vi "1mabsclass_1000dt.vi"() -> (0 "max jitter (uS)":dbl format="%.2f", 1 "mean time (uS)":dbl format="%.2f", 2 "standard deviation (uS)":dbl format="%.2f", 3 "execution histogram":T1(graph), 4 "Error":errorcluster, 5 "execution times (uS)":dbl[](graph))   [LabVIEW 2013]
uses:
  <vilib>/platform/TimedLoop/XDataNode/XDataNode.xnode
  <vilib>/Platform/TimedLoop/XDataNode/nitl_modes.ctl
  <vilib>/Platform/TimedLoop/XDataNode/XDNodeRunTimeDep.lvlib
  <vilib>/Platform/TimedLoop/XDataNode/wakeup.ctl
  <vilib>/Platform/TimedLoop/XDataNode/timing_clust.ctl
  absolute timing source/absolute usec timing source.lvclass
panel:
  out "act start":timestamp
  out "x-y":dbl
  out "current time":timestamp
  out "start":timestamp
  out "actual":dbl format="%#_32f"
  out "desired":dbl format="%#_32f"
  out "diff":dbl format="%#_32f"
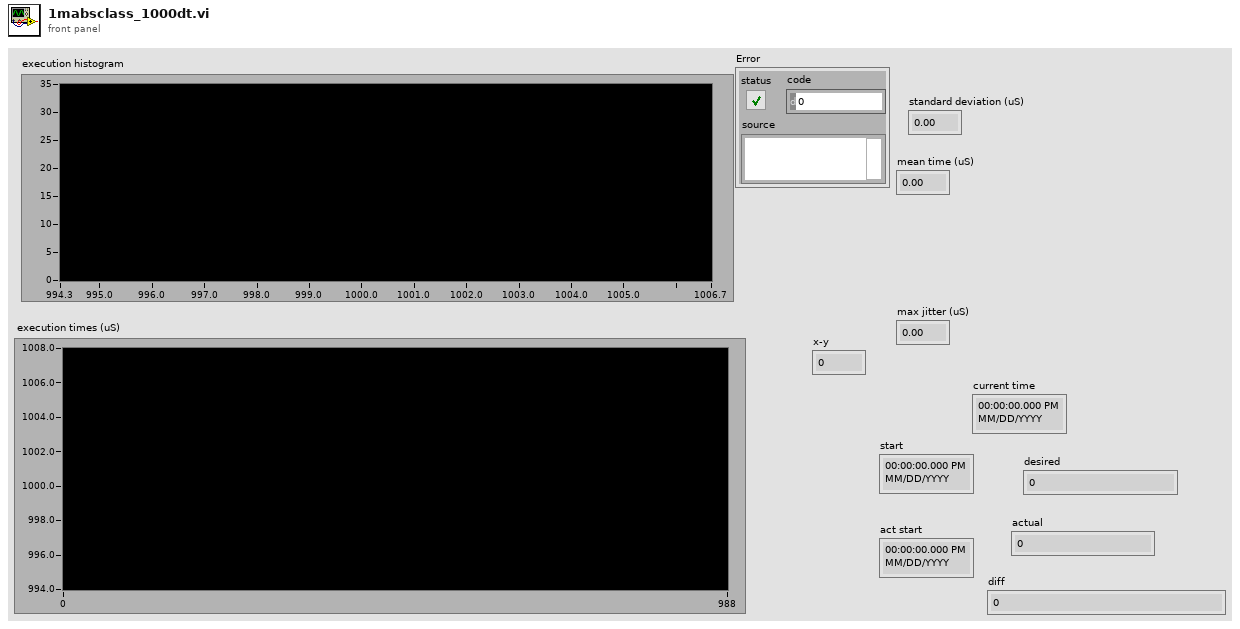
[diagram p1: front panel]
types:
  T1 = cluster{"X Values":dbl[], "Histogram: h(x)":i32[]}
  T2 = typedef "LVDateTimeRec.ctl" = cluster{"fractional second":dbl, "second":i32, "minute":i32, "hour":i32, "day of month":i32, "month":i32, "year":i32, "day of week":i32, "day of year":i32, "DST":i32}
  T3 = typedef "XDNodeRunTimeDep.lvlib/timing_clust.ctl" = cluster{"Expected End [f-1]":u64, "Actual End [f-1]":u64, "Finished Late? [f-1]":bool, "Expected End [i-1]":u64, "Actual End [i-1]":u64, "Finished Late? [i-1]":bool, "Expected Start [i]":u64, "Actual Start [i]":u64, "Expected Start [f]":u64, "Actual Start [f]":u64, "Source Name":string, "Structure Name":string, "Period":i64, "Deadline":i64, "Offset":i64, "Start":i64, "Priority":i32, "Timeout":i32, "Mode":T4, "Wakeup Reason":T5, "Error":errorcluster, "Source Type":string, "Secondary Source Type":string, "Global End Time":u64, "Global Start Time":u64, "Frame Duration":u64, "Iteration Duration":u64, "Assigned CPU":i32, "I/O Scan Engine Mode":u32}
  T4 = typedef "XDNodeRunTimeDep.lvlib/nitl_modes.ctl" = enum32{"No Change", "Process missed periods, maintain original phase", "Discard missed periods, maintain original phase", "Process missed periods, ignore original phase", "Discard missed periods, ignore original phase"}
  T5 = typedef "XDNodeRunTimeDep.lvlib/wakeup.ctl" = enum32{"Normal", "Aborted", "Asynchronous wakeup", "Timing source error", "Timed loop error", "Timeout"}
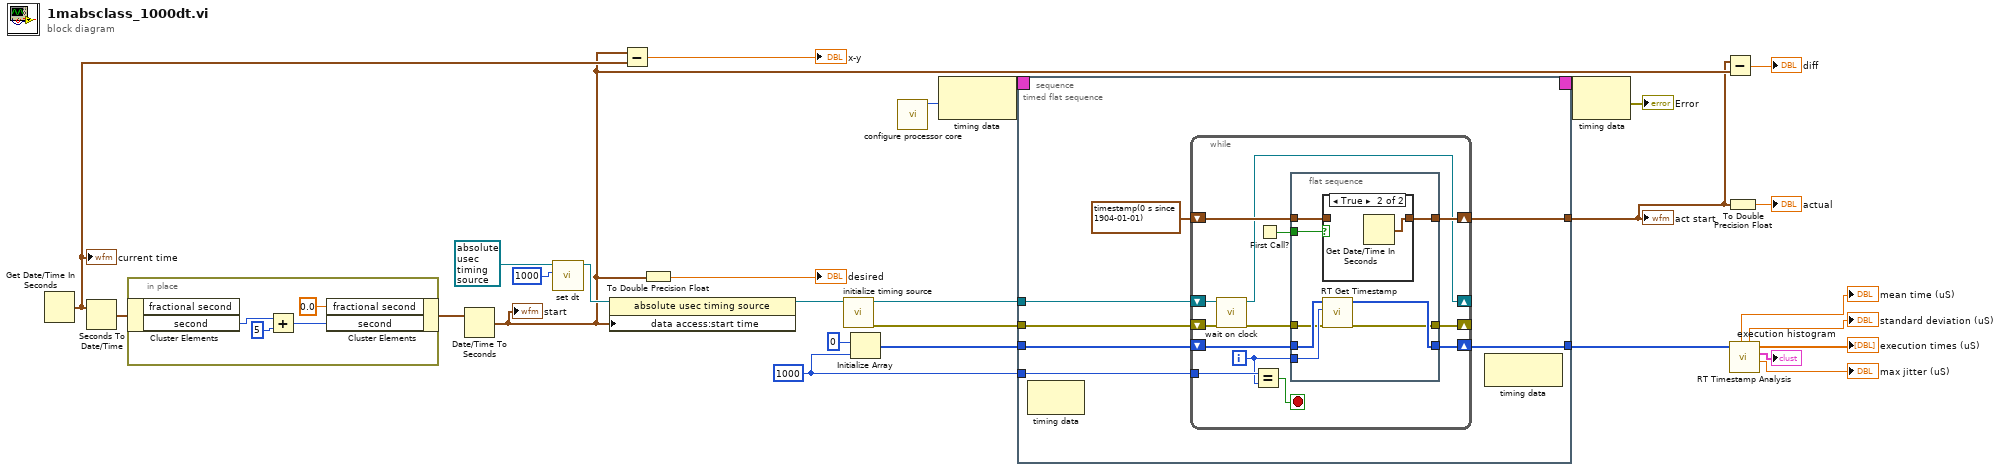
[diagram p0: block diagram]
diagram:
  w26 = 1000 ("x")
  n1 = Get Date/Time In Seconds() -> (seconds since 1Jan1904=w5:timestamp)
  "current time" <- w5
  n2 = Seconds To Date/Time(time stamp (now)=w5) -> (date time rec=w8:T2)  [unwired: 1 in]
  n3 = in-place {
    n4 = in-place-cluster #1(w8) -> ("second"=w31:i32)  [unwired: 1 out]
    n5 = Add(x=w31, y=5) -> (x+y=w29:i32)
    n6 = in-place-cluster #1("fractional second"=0.0, "second"=w29) -> (w7:T2)
  }
  n7 = Date/Time To Seconds(2:w7) -> (0:w2:timestamp)  [unwired: 1 in]
  "start" <- w2
  n8 = call "set dt.vi"("dt"=u32 1000, "timing source in"=refnum<class "absolute usec timing source.lvclass"> refnum ("absolute usec timing source.lvclass")) -> ("timing source out"=w14:refnum<class "absolute usec timing source.lvclass">)  [unwired: 9 in]
  n9 = property class="absolute usec timing source"(reference=w14, "data access:start time"=w2) -> (reference out=w3:refnum<class "absolute usec timing source.lvclass">)  [unwired: 1 in, 1 out]
  n10 = Subtract(x=w2, y=w5) -> (x-y=→"x-y":dbl)
  n11 = To Double Precision Float(number=w2) -> (double precision float=→"desired":dbl)
  n12 = call-dynamic "initialize timing source.vi"("timing source in"=w3) -> ("error out"=w12:errorcluster, "timing source out"=w13:refnum<class "absolute usec timing source.lvclass">)  [unwired: 9 in]
  n13 = Initialize Array(u64 0, w26) -> (w27:u64[])
  n14 = call "configure processor core.vi"() -> ("Processor"=w16:i32)  [unwired: 11 in]
  n15 = node-c288(w16) -> (w19:T3)
  n16 = timed-sequence {
    timing: w19 -> [_]
    timing-out: [_] -> w18
    tunnel: w26 -> [w38]
    tunnel: w27 -> [w37]
    tunnel: [w36] -> w25
    tunnel: w13 -> [w35]
    tunnel: w12 -> [w34]
    tunnel: [w33] -> w1
    n17 = timed-flat-sequence {
      tunnel: w38 -> [w45]
      tunnel: w37 -> [w44]
      tunnel: [w43] -> w36
      tunnel: w35 -> [w42]
      tunnel: w34 -> [w41]
      tunnel: [w39] -> w33
      n18 = node-c288() -> ()  [unwired: 1 in, 1 out]
      n19 = while {
        tunnel: w45 -> [w58]
        shift-right: [w56] -> w43
        shift-left: w44 -> [w57]
        shift-right: [w46] -> _
        shift-left: w42 -> [w52]
        shift-right: [w51] -> _
        shift-left: w41 -> [w50]
        shift-right: [w48] -> w39
        shift-left: timestamp(0 s since 1904-01-01) ("seconds since 1Jan1904") -> [w47]
        i -> [w54]
        stop <- w55 stop-if-true
        n20 = call-dynamic "wait on clock.vi"("error in"=w50, "timing source in"=w52) -> ("error out"=w53:errorcluster, "timing source out"=w46:refnum<class "absolute usec timing source.lvclass">)  [unwired: 7 in, 1 out]
        n21 = Equal?(x=w58, y=w54) -> (x = y?=w55:bool)
        n22 = First Call?() -> (First Call?: T/F=w49:bool)
        n23 = flat-sequence {
          tunnel: w57 -> [w66]
          tunnel: [w65] -> w56
          tunnel: w54 -> [w64]
          tunnel: w53 -> [w63]
          tunnel: [w62] -> w51
          tunnel: w49 -> [w61]
          tunnel: [w60] -> w48
          tunnel: w47 -> [w59]
          frame #0 {
            n24 = case shown="True" w61 {
              tunnel: [w67 w68] -> w60
              tunnel: w59 -> [w67 _]
              frame False {
              }
              frame True {
                n25 = Get Date/Time In Seconds() -> (seconds since 1Jan1904=w68:timestamp)
              }
            }
            n26 = call <vilib>:"RT Get Timestamp.vi"("error in (no error)"=w63, "iteration"=w64, "timestamp array in"=w66) -> ("error out"=w62:errorcluster, "timestamp array out"=w65:u64[])  [unwired: 7 in]
          }
        }
      }
      n27 = node-c288() -> ()  [unwired: 1 in, 1 out]
    }
  }
  "act start" <- w1
  n28 = node-c288(w18) -> (→"Error":errorcluster)
  n29 = Subtract(x=w1, y=w2) -> (x-y=→"diff":dbl)
  n30 = To Double Precision Float(number=w1) -> (double precision float=→"actual":dbl)
  n31 = call <vilib>:"RT Timestamp Analysis.vi"("timestamp array"=w25) -> ("max jitter (uS)"=→"max jitter (uS)":dbl, "execution histogram"=→"execution histogram":T1, "execution times (uS)"=→"execution times (uS)":dbl[], "standard deviation (uS)"=→"standard deviation (uS)":dbl, "mean time (uS)"=→"mean time (uS)":dbl)  [unwired: 5 in, 1 out]
